vi "ADSR Generator.vi"(8 "error in":errorcluster, 11 "FPGA VI Reference In":T1) -> (0 "error out":errorcluster)   [LabVIEW 2015]
uses:
  Controls/FPGA Reference.ctl
  Controls/ADSR State.ctl
  Controls/Application Data.vi
  <vilib>/rvi/interface/common/niFpgaWaitOnOcc.vi
  <vilib>/Utility/error.llb/Error Cluster From Error Code.vi
  <vilib>/rvi/errors/niLvFpgaAdjustHostInterfaceError.vi
  <vilib>/rvi/interface/nirviMethod/nirviMethod.xnode
  <vilib>/rvi/errors/niLvFpgaMergeErrorWithErrorCode.vi
  <vilib>/FPGAPlugInAG/Dynamic/niLvFpga_ConfigureFifo_Dynamic.vi
  <vilib>/FPGAPlugInAG/Dynamic/niLvFpga_StartFifo_Dynamic.vi
  <vilib>/FPGAPlugInAG/Dynamic/niLvFpga_WriteFifo_Dynamic.vi
panel:
  out "Gain2":dbl
  out "Gain Graph 2":dbl(graph)
  out "Waveform Chart":dbl[](graph)
  in  "Waveform":dbl[](array[numeric])
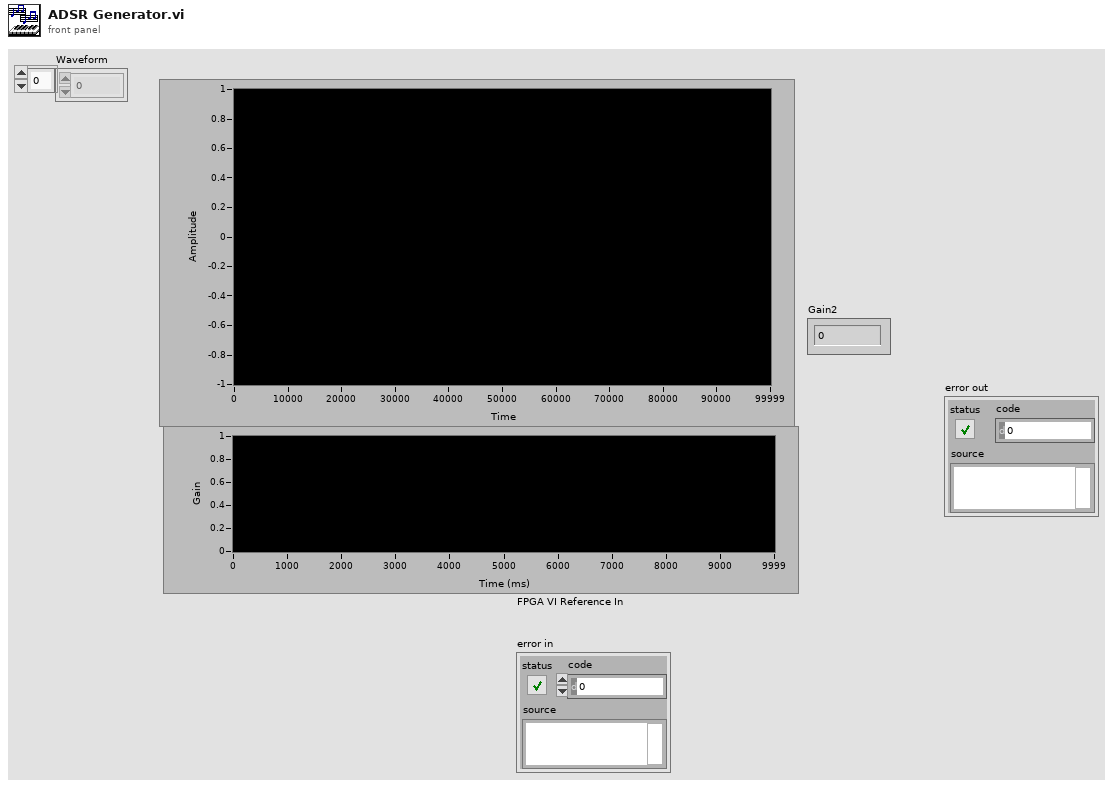
[diagram p1: front panel]
types:
  T1 = typedef "FPGA Reference.ctl" = refnum<k20>
  T2 = typedef "ADSR State.ctl" = enum16{"Attack", "Decay", "Sustain", "Release", "Idle"}
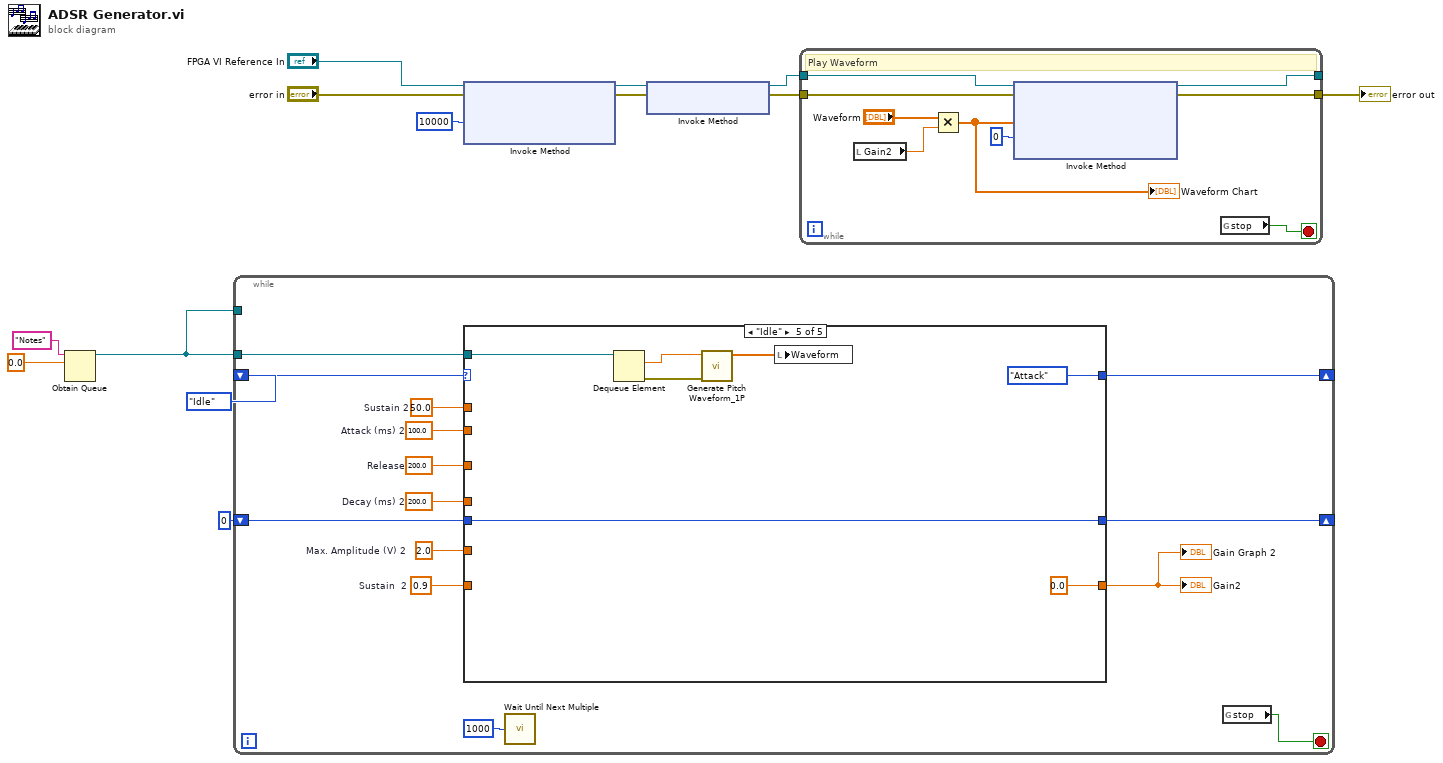
[diagram p0: block diagram]
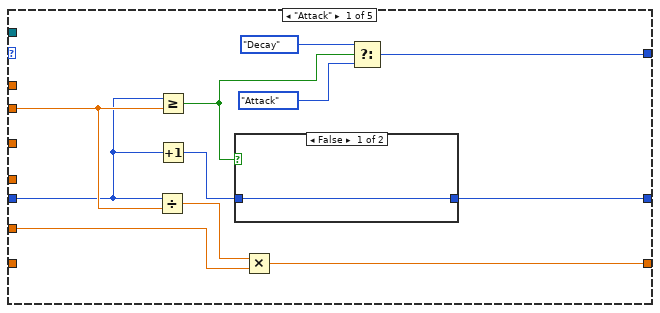
[diagram p2: hidden frame]
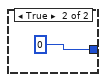
[diagram p3: hidden frame]
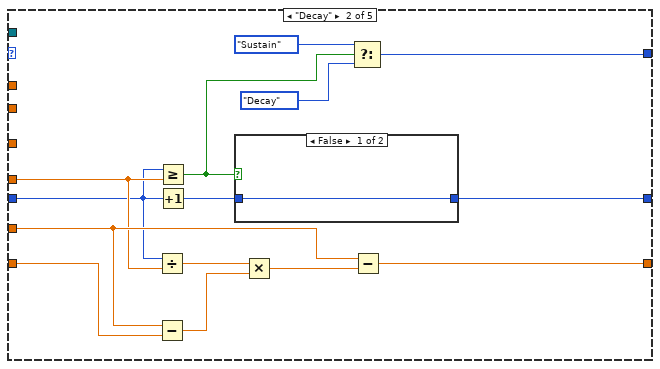
[diagram p4: hidden frame]
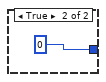
[diagram p5: hidden frame]
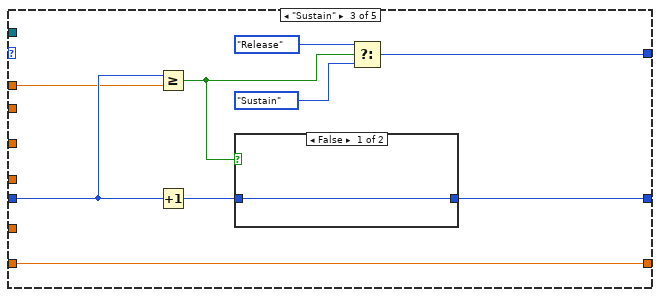
[diagram p6: hidden frame]
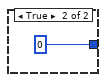
[diagram p7: hidden frame]
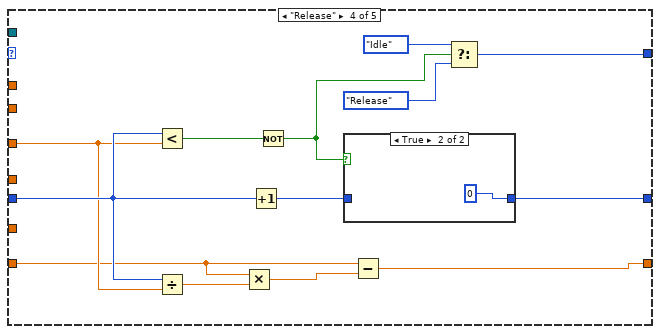
[diagram p8: hidden frame]
diagram:
  n1 = Obtain Queue(name (unnamed)="Notes", element data type=0.0) -> (queue out=w1:refnum<queue>)  [unwired: 3 in, 2 out]
  n2 = while {
    shift-right: [w26] -> _
    shift-left: ADSR_State."Idle" -> [w27]
    shift-right: [w23] -> _
    shift-left: 0 -> [w24]
    tunnel: w1 -> [w21]
    tunnel: w1 -> [_]
    stop <- w14 stop-if-true
    w15 = 200.0  # Release
    w16 = 50.0  # Sustain 2
    w17 = 200.0  # Decay (ms) 2
    w18 = 100.0  # Attack (ms) 2
    w20 = 0.9  # Sustain  2
    w19 = 2.0  # Max. Amplitude (V) 2
    n3 = case shown="\"Idle\"" w27 {
      tunnel: w20 -> [_ w54 w57 w73 _]
      tunnel: w19 -> [w37 w51 _ _ _]
      tunnel: w18 -> [w32 _ _ _ _]
      tunnel: w17 -> [_ w45 _ _ _]
      tunnel: w16 -> [_ _ w58 _ _]
      tunnel: w15 -> [_ _ _ w76 _]
      tunnel: w24 -> [w30 w43 w59 w77 w88]
      tunnel: [w36 w49 w57 w72 0.0 ("Sustain (%) 2")] -> w22
      tunnel: [w33 w46 w61 w71 ADSR_State."Attack"] -> w26
      tunnel: [w29 w41 w64 w79 w88] -> w23
      tunnel: w21 -> [_ _ _ _ w83]
      frame "Attack" {
        n4 = Divide(x=w30, y=w32) -> (x/y=w38:dbl)
        n5 = Greater Or Equal?(x=w30, y=w32) -> (x >= y?=w28:bool)
        n6 = Increment(x=w30) -> (x+1=w31:i32)
        n7 = case shown="False" w28 {
          tunnel: w31 -> [w39 _]
          tunnel: [w39 0] -> w29
          frame False {
          }
          frame True {
          }
        }
        n8 = Multiply(x=w38, y=w37) -> (x*y=w36:dbl)
        n9 = Select(t=ADSR_State."Decay", s=w28, f=ADSR_State."Attack") -> (s? t:f=w33:T2)
      }
      frame "Decay" {
        n10 = Divide(x=w43, y=w45) -> (x/y=w53:dbl)
        n11 = Subtract(x=w51, y=w54) -> (x-y=w52:dbl)
        n12 = Greater Or Equal?(x=w43, y=w45) -> (x >= y?=w44:bool)
        n13 = Increment(x=w43) -> (x+1=w42:i32)
        n14 = case shown="False" w44 {
          tunnel: w42 -> [w55 _]
          tunnel: [w55 0] -> w41
          frame False {
          }
          frame True {
          }
        }
        n15 = Multiply(x=w53, y=w52) -> (x*y=w50:dbl)
        n16 = Select(t=ADSR_State."Sustain", s=w44, f=ADSR_State."Decay") -> (s? t:f=w46:T2)
        n17 = Subtract(x=w51, y=w50) -> (x-y=w49:dbl)
      }
      frame "Sustain" {
        n18 = Greater Or Equal?(x=w59, y=w58) -> (x >= y?=w60:bool)
        n19 = Increment(x=w59) -> (x+1=w65:i32)
        n20 = case shown="False" w60 {
          tunnel: w65 -> [w66 _]
          tunnel: [w66 0] -> w64
          frame False {
          }
          frame True {
          }
        }
        n21 = Select(t=ADSR_State."Release", s=w60, f=ADSR_State."Sustain") -> (s? t:f=w61:T2)
      }
      frame "Release" {
        n22 = Less?(x=w77, y=w76) -> (x < y?=w78:bool)
        n23 = Divide(x=w77, y=w76) -> (x/y=w75:dbl)
        n24 = Multiply(x=w73, y=w75) -> (x*y=w74:dbl)
        n25 = Increment(x=w77) -> (x+1=w80:i32)
        n26 = Not(x=w78) -> (.not. x?=w68:bool)
        n27 = case shown="True" w68 {
          tunnel: w80 -> [w81 _]
          tunnel: [w81 0] -> w79
          frame False {
          }
          frame True {
          }
        }
        n28 = Subtract(x=w73, y=w74) -> (x-y=w72:dbl)
        n29 = Select(t=ADSR_State."Idle", s=w68, f=ADSR_State."Release") -> (s? t:f=w71:T2)
      }
      frame "Idle" {
        n30 = Dequeue Element(queue=w83) -> (element=w86:dbl, error out=w84:errorcluster)  [unwired: 2 in, 2 out]
        n31 = call "Generate Pitch Waveform_1P.vi"("Error In"=w84, "Pitch Frequency"=w86) -> ("Pitch Waveform"=w87:dbl[])  [unwired: 8 in, 1 out]
        n32 = local write "Waveform"(w87) -> ()
      }
    }
    "Gain2" <- w22
    "Gain Graph 2" <- w22
    n33 = call "Wait Until Next Multiple"("Count(uSec)"=u32 1000) -> ()  [unwired: 1 out]
    n34 = global read "Application Data.vi" "stop"() -> (w14:bool)
  }
  n35 = xnode "Invoke Method"("FPGA VI Reference In"="FPGA VI Reference In", "error in"="error in", "Requested Depth"=u32 10000) -> ("FPGA VI Reference Out"=w9:T1, "error out"=w10:errorcluster)  [unwired: 1 out]
  n36 = xnode "Invoke Method"("FPGA VI Reference In"=w9, "error in"=w10) -> ("FPGA VI Reference Out"=w8:T1, "error out"=w5:errorcluster)
  n37 = while {
    tunnel: w8 -> [w96]
    tunnel: [w95] -> w4
    tunnel: [w94] -> _
    tunnel: w5 -> [w92]
    stop <- w91 stop-if-true
    # "Play Waveform"
    n38 = local read "Gain2"() -> (w90:dbl)
    n39 = Multiply(x="Waveform", y=w90) -> (x*y=w98:dbl[])
    "Waveform Chart" <- w98
    n40 = xnode "Invoke Method"("FPGA VI Reference In"=w96, "error in"=w92, "Data"=w98, "Timeout (ms)"=0) -> ("FPGA VI Reference Out"=w94:T1, "error out"=w95:errorcluster)  [unwired: 1 out]
    n41 = global read "Application Data.vi" "stop"() -> (w91:bool)
  }
  "error out" <- w4
